vi "8.vi"() -> ()   [LabVIEW 2021]
panel:
  out "Cluster":cluster{u64[], u64}
  in  "Number of Consecutive digits":i32=1 min=1
  out "size(s)":i32
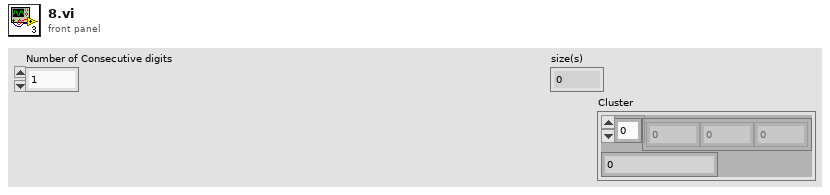
[diagram p1: front panel]
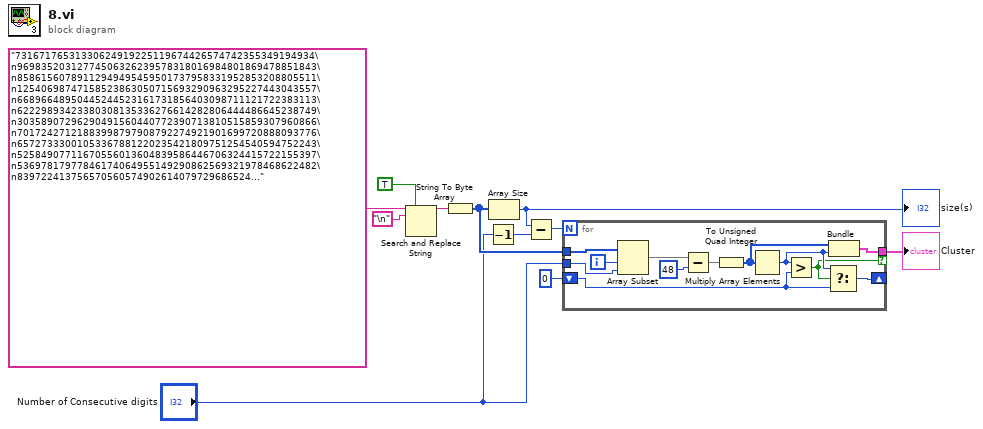
[diagram p0: block diagram]
diagram:
  n1 = Search and Replace String(replace all?=TRUE ("replace all? (F)"), input string="73167176531330624919225119674426574742355349194934\n96983520312774506326239578318016984801869478851843\n85861560789112949495459501737958331952853208805511\n12540698747158523863050715693290963295227443043557\n66896648950445244523161731856403098711121722383113\n62229893423380308135336276614282806444486645238749\n30358907296290491560440772390713810515859307960866\n70172427121883998797908792274921901699720888093776\n65727333001053367881220235421809751254540594752243\n52584907711670556013604839586446706324415722155397\n53697817977846174064955149290862569321978468622482\n83972241375657056057490261407972968652414535100474\n82166370484403199890008895243450658541227588666881\n16427171479924442928230863465674813919123162824586\n17866458359124566529476545682848912883142607690042\n24219022671055626321111109370544217506941658960408\n07198403850962455444362981230987879927244284909188\n84580156166097919133875499200524063689912560717606\n05886116467109405077541002256983155200055935729725\n71636269561882670428252483600823257530420752963450", search string="\n") -> (result string=w8:string)  [unwired: 5 in, 3 out]
  n2 = String To Byte Array(string=w8) -> (unsigned byte array=w4:u8[])
  n3 = Decrement(x="Number of Consecutive digits") -> (x-1=w5:i32)
  n4 = Array Size(array=w4) -> (size(s)=w6:i32)
  "size(s)" <- w6
  n5 = Subtract(x=w6, y=w5) -> (x-y=w7:i32)
  n6 = for {
    N: w7 -> [_]
    tunnel: w4 -> [w23]
    tunnel: "Number of Consecutive digits" -> [w21]
    shift-right: [w20] -> _
    shift-left: u64 0 -> [w19]
    tunnel: [w18] -> w1 if=w12
    i -> [w22]
    n7 = Array Subset(array=w23, index=w22, length=w21) -> (w15:u8[])
    n8 = Subtract(x=w15, y=u8 48) -> (x-y=w14:u8[])
    n9 = To Unsigned Quad Integer(1:w14) -> (0:w13:u64[])
    n10 = Multiply Array Elements(1:w13) -> (0:w17:u64)
    n11 = Greater?(x=w17, y=w19) -> (0:w12:bool)
    n12 = Select(t=w17, s=w12, f=w19) -> (s? t:f=w20:u64)
    n13 = Bundle(w13, w17) -> (w18:cluster{u64[], u64})  [unwired: 1 in]
  }
  "Cluster" <- w1
